vi "AD5933_GetTemp (NI-845x I2C)(SubVI).vi"(8 "error in (no error)":errorcluster, 11 "NI-845x Config for I2C (out) in":T3) -> (0 "error out":errorcluster, 2 "Temperature":dbl, 3 "NI-845x Config for I2C (out) out":T3)   [LabVIEW 2017]
uses:
  <vilib>/ni845x/ni845x.llb/ni845xI2cConfiguration.ctl
  <vilib>/ni845x/ni845x.llb/ni845xControl.ctl
  TypeDefs/AD5933_CommandCodes.ctl
  TypeDefs/AD5933_Registers.ctl
  <vilib>/MakerHub/Toolbox/LMH-Toolbox.lvlib
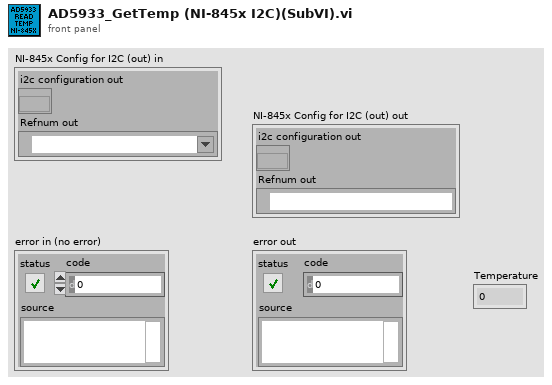
[diagram p1: front panel]
types:
  T1 = typedef "ni845xI2cConfiguration.ctl" = refnum<k20>
  T2 = typedef "ni845xControl.ctl" = refnum<k21>
  T3 = cluster{"i2c configuration out":T1, "Refnum out":T2}
  T4 = typedef "AD5933_CommandCodes.ctl" = u8
  T5 = typedef "AD5933_Registers.ctl" = u8
  T6 = cluster{"Valid temperature measurement":bool, "Valid real/imaginary data":bool, "Frequency sweep complete":bool}
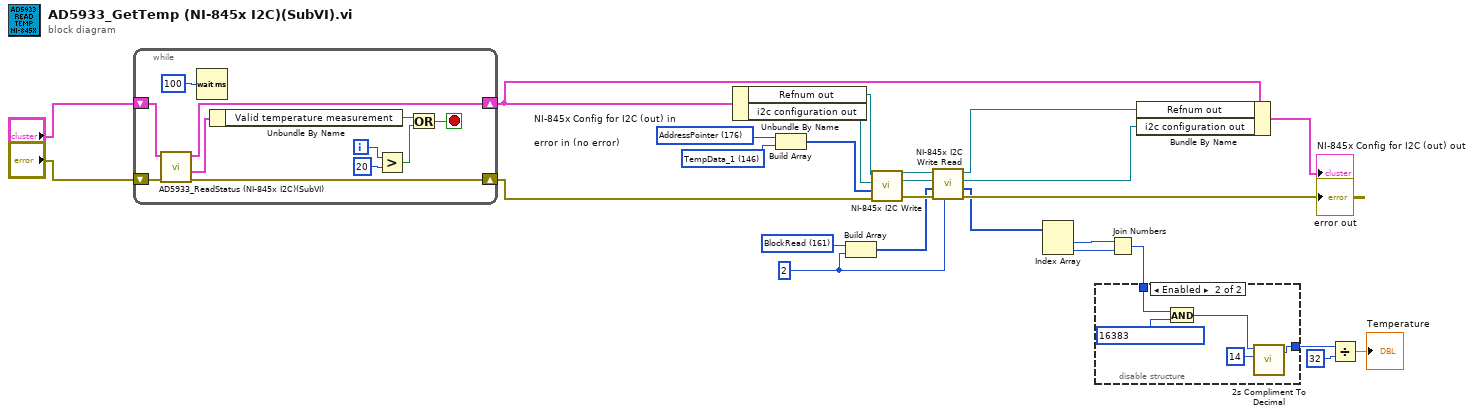
[diagram p0: block diagram]
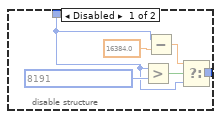
[diagram p2: hidden frame]
diagram:
  w10 = 2
  w16 = T4 161 items=["BlockWrite"=160, "BlockRead"=161, "AddressPointer"=176] ("CommandCodes")
  w17 = T5 146 items=["Control_1"=128, "Control_0"=129, "StartFeq_2"=130, "StartFeq_1"=131, "StartFeq_0"=132, "FreqInc_2"=133, "FreqInc_1"=134, "FreqInc_0"=135, "NumOfInc_1"=136, "NumOfInc_0"=137, "NumOfSetCycl_1"=138, "NumOfSetCycl_0"=139, "Status"=143, "TempData_1"=146, "TempData_0"=147, "RealData_1"=148, "RealData_0"=149, "ImagData_1"=150, "ImagData_0"=151] ("Register")
  w18 = T4 176 items=["BlockWrite"=160, "BlockRead"=161, "AddressPointer"=176] ("CommandCodes")
  n1 = while {
    shift-right: [w35] -> w2
    shift-left: "NI-845x Config for I2C (out) in" -> [w37]
    shift-right: [w34] -> w1
    shift-left: "error in (no error)" -> [w36]
    i -> [w28]
    stop <- w30 stop-if-true
    n2 = call "AD5933_ReadStatus (NI-845x I2C)(SubVI).vi"("error in"=w36, "NI-845x Config for I2C (in)"=w37) -> ("error out"=w34:errorcluster, "Status Info"=w33:T6, "NI-845x Config for I2C (out)"=w35:T3)  [unwired: 6 in]
    n3 = Wait (ms)(milliseconds to wait=u32 100) -> ()  [unwired: 1 out]
    n4 = Unbundle By Name(w33) -> ("Valid temperature measurement"=w31:bool)
    n5 = Greater?(x=w28, y=20) -> (0:w29:bool)
    n6 = Or(x=w31, y=w29) -> (x .or. y?=w30:bool)
  }
  n7 = Unbundle By Name(w2) -> ("Refnum out"=w19:T2, "i2c configuration out"=w20:T1)
  n8 = Build Array(w18, w17) -> (w24:T5[])
  n9 = Build Array(w16, w10) -> (w15:i32[])
  n10 = call <vilib>:"NI-845x I2C Write.vi"("error in (no error)"=w1, "write data"=w24, "i2c configuration in"=w20, "device reference in"=w19) -> ("error out"=w23:errorcluster, "i2c configuration out"=w22:T1, "device reference out"=w21:T2)  [unwired: 5 in]
  n11 = call <vilib>:"NI-845x I2C Write Read.vi"("num bytes to read"=w10, "error in (no error)"=w23, "write data"=w15, "i2c configuration in"=w22, "device reference in"=w21) -> ("error out"=→"error out":errorcluster, "read data"=w9:u8[], "i2c configuration out"=w13:T1, "device reference out"=w14:T2)  [unwired: 3 in]
  n12 = Index Array(array=w9) -> (element #1=w12:u8, element #2=w11:u8)  [unwired: 2 in]
  n13 = Join Numbers(hi=w12, lo=w11) -> ((hi.lo)=w5:u16)
  n14 = disable-structure shown="Enabled" {
    disable-tunnel: [w43 w45] -> w6
    disable-tunnel: w5 -> [w38 w48]
    frame Disabled {
      n15 = Greater?(x=w38, y=u16 8191 ("Numeric")) -> (0:w40:bool)
      n16 = Subtract(x=w38, y=16384.0) -> (x-y=w41:dbl)
      n17 = Select(t=w41, s=w40, f=w38) -> (s? t:f=w43:dbl)
    }
    frame Enabled {
      n18 = And(x=w48, y=u16 16383 ("Numeric")) -> (x .and. y?=w44:u16)
      n19 = call <vilib>:"2s Compliment To Decimal.vi"("Bit Width (8)"=14, "2s Comp Number"=w44) -> ("Decimal Number"=w45:i32)  [unwired: 3 in]
    }
  }
  n20 = Bundle By Name(cluster=w2, "Refnum out"=w14, "i2c configuration out"=w13) -> (→"NI-845x Config for I2C (out) out":T3)
  n21 = Divide(x=w6, y=u16 32) -> (x/y=→"Temperature":dbl)
